vi "Get Pin Map Context.vi"(8 "error in":errorcluster, 11 "measure call context in":refnum<class "Measure Call Context.lvclass">) -> (0 "error out":errorcluster, 2 "pin map context":T1, 3 "measure call context out":refnum<class "Measure Call Context.lvclass">)   [LabVIEW 2020, in "MeasurementLink Measurement Server.lvlib" / "Measure Call Context.lvclass"]
doc: "Gets the pin map context for the measurement. The pin map context is used to reserve and unreserve sessions using the session management client."
uses:
  Measure Call Context.lvclass
  Helpers/TypeDefs/Pin Map Context.ctl
  Measure Call Context.lvclass/Measure Call Context.ctl
  MeasurementLink Measurement Server.lvlib
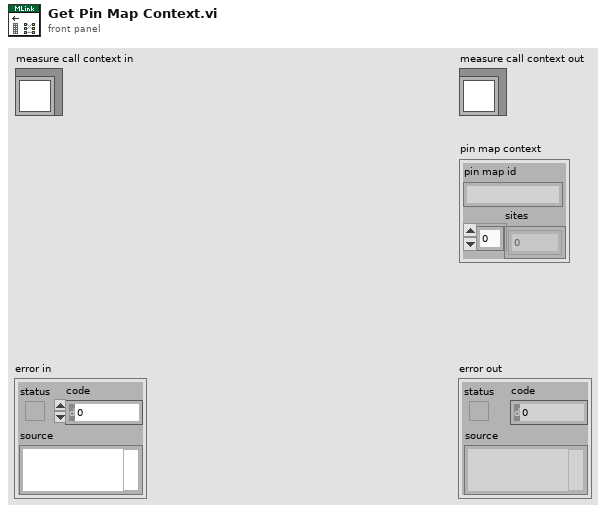
[diagram p1: front panel]
types:
  T1 = typedef "MeasurementLink Measurement Server.lvlib/Pin Map Context.ctl" = cluster{"pin map id":string, "sites":i32[]}
  T2 = typedef "MeasurementLink Measurement Server.lvlib/Measure Call Context.lvclass/Data.ctl" = cluster{"pin map context":T3, "gRPC ID":T4, "measurement service":refnum<class "IMeasurement Service.lvclass">, "measurement plugin service":refnum<class "Measurement Plugin Service.lvclass">, "reserved session infos":set{T5}}
  T3 = typedef "MeasurementLink Measurement Server.lvlib/PinMapContext.ctl" = cluster{"pin map id":string, "sites":i32[]}
  T4 = typedef "grpc-lvsupport-release.lvlib/grpcId.ctl" = u64
  T5 = typedef "MeasurementLink Session Management Client.lvlib/ni_measurementlink_sessionmanagement_v1_SessionInformation.ctl" = cluster{"session":T6, "resource_name":string, "channel_list":string, "instrument_type_id":string, "session_exists":bool, "channel_mappings":T7[]}
  T6 = typedef "MeasurementLink Session Management Client.lvlib/nidevice_grpc_Session.ctl" = cluster{"name":string}
  T7 = typedef "MeasurementLink Session Management Client.lvlib/ni_measurementlink_sessionmanagement_v1_ChannelMapping.ctl" = cluster{"pin_or_relay_name":string, "site":i32, "channel":string}
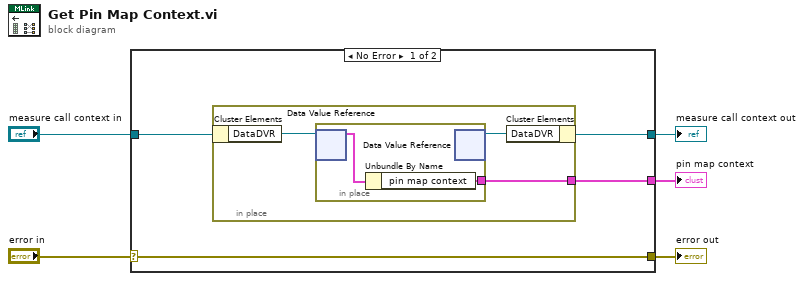
[diagram p0: block diagram]
diagram:
  n1 = case shown="No Error" "error in" {
    selector: "error in" -> [w9 w15]
    tunnel: [w9 w15] -> w4
    tunnel: [w7 w16] -> w2
    tunnel: "measure call context in" -> [w8 w16]
    tunnel: [w6 _] -> w1
    frame No Error {
      n2 = in-place {
        in-place-border: [w10] -> w6
        n3 = in-place-cluster #1(w8) -> ("DataDVR"=w12:refnum<data-value>)
        n4 = in-place {
          in-place-border: [w13] -> w10
          n5 = in-place-dvr #2(w12) -> (w14:T2)  [unwired: 1 out]
          n6 = Unbundle By Name(w14) -> ("pin map context"=w13:T3)
          n7 = in-place-dvr #2() -> (w11:refnum<data-value>)  [unwired: 1 in, 1 out]
        }
        n8 = in-place-cluster #1("DataDVR"=w11) -> (w7:refnum<class "Measure Call Context.lvclass">)
      }
    }
    frame Error {
    }
  }
  "error out" <- w4
  "measure call context out" <- w2
  "pin map context" <- w1
